vi "Read Capabilities.vi"(8 "error in (no error)":errorcluster, 11 "SLSC Switch in":refnum<class "SLSC Switch.lvclass">) -> (0 "error out":errorcluster, 2 "capabilities":string)   [LabVIEW 2015, in "SLSC Switch.lvclass"]
uses:
  SLSC Switch.lvclass
  SLSC Switch.lvclass/SLSC Switch.ctl
  <vilib>/SLSC/Initialize Session with NVMEM Areas.vi
  <vilib>/SLSC/Close Session.vi
  <vilib>/SLSC/SLSC.lvlib
  <resource>/objmgr/slsc.rc
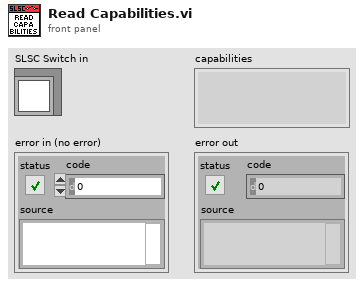
[diagram p1: front panel]
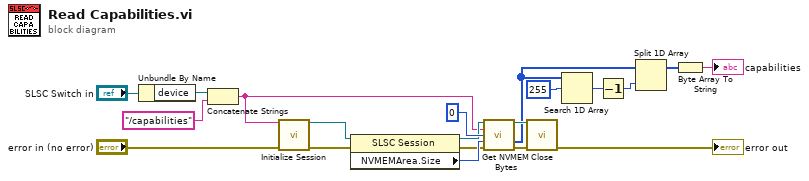
[diagram p0: block diagram]
diagram:
  n1 = Unbundle By Name("SLSC Switch in") -> ("device"=w16:refnum<k21>)
  n2 = Concatenate Strings(w16, "/capabilities" ("string")) -> (w8:string)
  n3 = call-poly <vilib>:"Initialize Session.vi"("NVMEM areas"=w8, "error in (no error)"="error in (no error)") -> ("session out"=w9:refnum<k21>, "error out"=w10:errorcluster)  [unwired: 12 in]
  n4 = property class="SLSC Session"(reference=w9, error in=w10) -> (reference out=w13:refnum<k21>, error out=w12:errorcluster, "NVMEMArea.Size"=w15:u32)
  n5 = call <vilib>:"Get NVMEM Bytes.vi"("session in"=w13, "NVMEM area"=w8, "data address"=u32 0, "data size"=w15, "error in (no error)"=w12) -> ("session out"=w7:refnum<k21>, "data out"=w4:u8[], "error out"=w6:errorcluster)  [unwired: 6 in, 2 out]
  n6 = call-poly <vilib>:"Close.vi"("session in"=w7, "error in (no error)"=w6) -> ("error out"=→"error out":errorcluster)  [unwired: 13 in]
  n7 = Search 1D Array(1D array=w4, element=u8 255) -> (index of element=w2:i32)  [unwired: 1 in]
  n8 = Decrement(x=w2) -> (x-1=w1:i32)
  n9 = Split 1D Array(array=w4, index=w1) -> (first subarray=w3:u8[])  [unwired: 1 out]
  n10 = Byte Array To String(unsigned byte array=w3) -> (string=→"capabilities":string)
